vi "sub_SparePinZoneCheck.vi"(8 "핀간격":dbl=40.0, 10 "Particle Reports (Pixels)":T1(array[cluster])=[{"Area"=385.0, "Number of Holes"=0.0, "Bounding Rect"={"Left"=657.0, "Top"=541.0, "Right"=674.0, "Bottom"=575.0}, "Center of Mass"={"X"=664.9506493506493, "Y"=559.8831168831168}, "Orientation"=90.17449143861148, "Dimensions"={"Width"=17.0, "Height"=34.0}}], 11 "참조 번호 입력":T2=refnum) -> (2 "숫자형":dbl=665.5, 3 "참조 번호 출력":T2)   [LabVIEW 2014]
uses:
  <vilib>/vision/Image Controls.llb/IMAQ Image.ctl
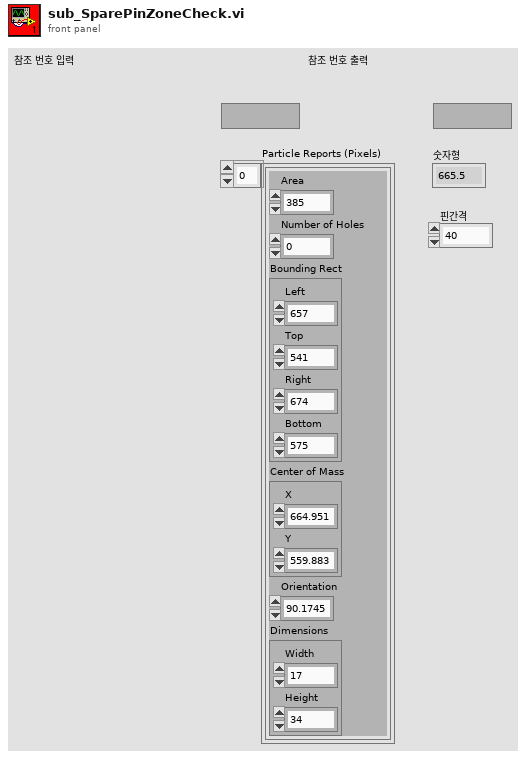
[diagram p1: front panel]
types:
  T1 = cluster{"Area":dbl, "Number of Holes":dbl, "Bounding Rect":cluster{"Left":dbl, "Top":dbl, "Right":dbl, "Bottom":dbl}, "Center of Mass":cluster{"X":dbl, "Y":dbl}, "Orientation":dbl, "Dimensions":cluster{"Width":dbl, "Height":dbl}}[]
  T2 = typedef "IMAQ Image.ctl" = refnum<image>
  T3 = cluster{"Area":dbl, "Number of Holes":dbl, "Bounding Rect":cluster{"Left":dbl, "Top":dbl, "Right":dbl, "Bottom":dbl}, "Center of Mass":cluster{"X":dbl, "Y":dbl}, "Orientation":dbl, "Dimensions":cluster{"Width":dbl, "Height":dbl}}
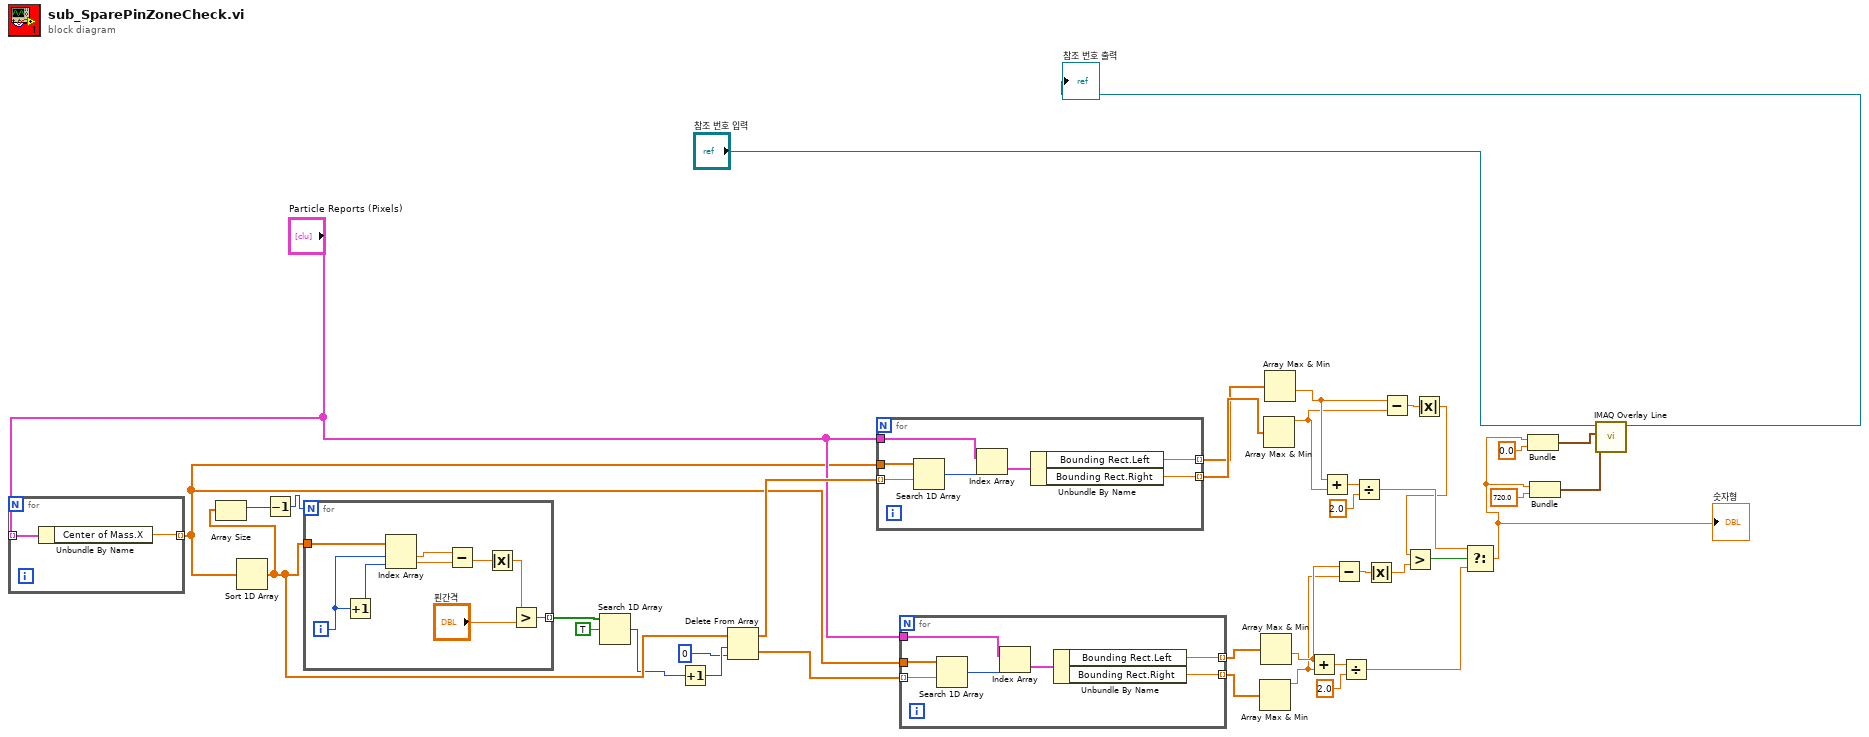
[diagram p0: block diagram]
diagram:
  n1 = for {
    tunnel: "Particle Reports (Pixels)" -> [w40] mode=indexing
    tunnel: [w39] -> w12 mode=indexing
    n2 = Unbundle By Name(w40) -> ("Center of Mass.X"=w39:dbl)
  }
  n3 = Sort 1D Array(array=w12) -> (sorted array=w6:dbl[])
  n4 = Array Size(array=w6) -> (size(s)=w1:i32)
  n5 = Decrement(x=w1) -> (x-1=w2:i32)
  n6 = for {
    N: w2 -> [_]
    tunnel: w6 -> [w49]
    tunnel: [w42] -> w3 mode=indexing
    i -> [w48]
    n7 = Increment(x=w48) -> (x+1=w47:i32)
    n8 = Index Array(array=w49, index #1=w48, index #2=w47) -> (element #1=w46:dbl, element #2=w45:dbl)
    n9 = Subtract(x=w46, y=w45) -> (x-y=w44:dbl)
    n10 = Absolute Value(x=w44) -> (abs(x)=w43:dbl)
    n11 = Greater?(x=w43, y="핀간격") -> (0:w42:bool)
  }
  n12 = Search 1D Array(1D array=w3, element=TRUE ("원소")) -> (index of element=w5:i32)  [unwired: 1 in]
  n13 = Increment(x=w5) -> (x+1=w8:i32)
  n14 = Delete From Array(array=w6, length=w8, index=0 ("인덱스")) -> (deleted portion=w11:dbl[], array with subset deleted=w38:dbl[])
  n15 = for {
    tunnel: w38 -> [w56] mode=indexing
    tunnel: w12 -> [w55]
    tunnel: "Particle Reports (Pixels)" -> [w54]
    tunnel: [w51] -> w9 mode=indexing
    tunnel: [w50] -> w10 mode=indexing
    n16 = Search 1D Array(1D array=w55, element=w56) -> (index of element=w53:i32)  [unwired: 1 in]
    n17 = Index Array(array=w54, index=w53) -> (element=w52:T3)
    n18 = Unbundle By Name(w52) -> ("Bounding Rect.Left"=w51:dbl, "Bounding Rect.Right"=w50:dbl)
  }
  n19 = for {
    tunnel: w11 -> [w63] mode=indexing
    tunnel: w12 -> [w62]
    tunnel: "Particle Reports (Pixels)" -> [w61]
    tunnel: [w58] -> w14 mode=indexing
    tunnel: [w57] -> w15 mode=indexing
    n20 = Search 1D Array(1D array=w62, element=w63) -> (index of element=w60:i32)  [unwired: 1 in]
    n21 = Index Array(array=w61, index=w60) -> (element=w59:T3)
    n22 = Unbundle By Name(w59) -> ("Bounding Rect.Left"=w58:dbl, "Bounding Rect.Right"=w57:dbl)
  }
  n23 = Array Max & Min(array=w15) -> (max value=w29:dbl)  [unwired: 3 out]
  n24 = Array Max & Min(array=w14) -> (min value=w30:dbl)  [unwired: 3 out]
  n25 = Array Max & Min(array=w10) -> (max value=w25:dbl)  [unwired: 3 out]
  n26 = Array Max & Min(array=w9) -> (min value=w26:dbl)  [unwired: 3 out]
  n27 = Add(x=w30, y=w29) -> (x+y=w19:dbl)
  n28 = Add(x=w26, y=w25) -> (x+y=w16:dbl)
  n29 = Subtract(x=w30, y=w29) -> (x-y=w28:dbl)
  n30 = Divide(x=w19, y=2.0) -> (x/y=w35:dbl)
  n31 = Divide(x=w16, y=2.0) -> (x/y=w34:dbl)
  n32 = Absolute Value(x=w28) -> (abs(x)=w32:dbl)
  n33 = Subtract(x=w26, y=w25) -> (x-y=w27:dbl)
  n34 = Absolute Value(x=w27) -> (abs(x)=w31:dbl)
  n35 = Greater?(x=w31, y=w32) -> (0:w33:bool)
  n36 = Select(t=w34, s=w33, f=w35) -> (s? t:f=w37:dbl)
  "숫자형" <- w37
  n37 = Bundle(w37, "y"=0.0) -> (w20:cluster{dbl, "y":dbl})  [unwired: 1 in]
  n38 = Bundle(w37, "y"=720.0) -> (w23:cluster{dbl, "y":dbl})  [unwired: 1 in]
  n39 = call "IMAQ Overlay Line"("End Point"=w23, "Start Point"=w20, "Image"="참조 번호 입력") -> ("Image Out"=→"참조 번호 출력":T2)  [unwired: 7 in, 1 out]
